vi "Create Custom Color Table.vi"(0 "Colors []":u32[](array[colorbox]), 1 "Size (256)":i32=256) -> (2 "Color Tbl":u32[](array[numeric]), 3 "R []":u8[](array[numeric]), 4 "G []":u8[](array[numeric]), 5 "B []":u8[](array[numeric]))   [LabVIEW 2016, in "graph_utilities.lvclass"]
doc: "Wire an array of colors to Color []. This VI will interpolate between the colors and return a R,G,B, and Color Table arrays."
uses:
  graph_utilities.lvclass
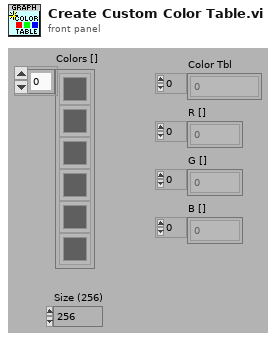
[diagram p1: front panel]
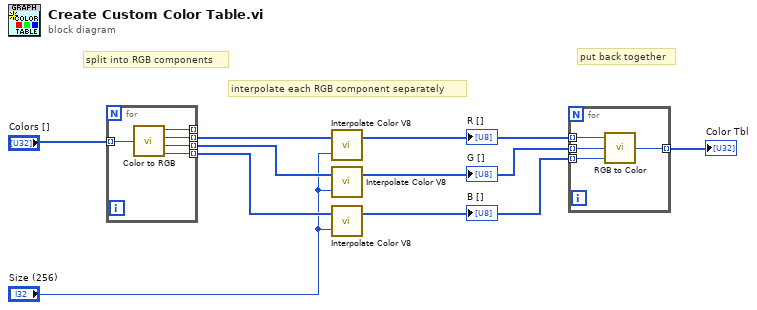
[diagram p0: block diagram]
diagram:
  # "put back together"
  # "interpolate each RGB component separately"
  # "split into RGB components"
  n1 = for {
    tunnel: "Colors []" -> [w14] mode=indexing
    tunnel: [w13] -> w9 mode=indexing
    tunnel: [w12] -> w7 mode=indexing
    tunnel: [w11] -> w6 mode=indexing
    tunnel: [w10] -> _ mode=indexing
    n2 = call <vilib>:"Color to RGB.vi"("Color"=w14) -> ("Resolved Color"=w10:u32, "R"=w13:u8, "G"=w12:u8, "B"=w11:u8)
  }
  n3 = call "Interpolate Color V8.vi"("Size (256)"="Size (256)", "Colors in"=w9) -> ("Colors out"=w4:u8[])  [unwired: 1 in]
  "R []" <- w4
  n4 = call "Interpolate Color V8.vi"("Size (256)"="Size (256)", "Colors in"=w7) -> ("Colors out"=w3:u8[])  [unwired: 1 in]
  "G []" <- w3
  n5 = call "Interpolate Color V8.vi"("Size (256)"="Size (256)", "Colors in"=w6) -> ("Colors out"=w5:u8[])  [unwired: 1 in]
  "B []" <- w5
  n6 = for {
    tunnel: w4 -> [w18] mode=indexing
    tunnel: w3 -> [w17] mode=indexing
    tunnel: w5 -> [w16] mode=indexing
    tunnel: [w15] -> w1 mode=indexing
    n7 = call <vilib>:"RGB to Color.vi"("B"=w16, "G"=w17, "R"=w18) -> ("Color"=w15:u32)
  }
  "Color Tbl" <- w1
